vi "linx_analog_okuma_deneme2.vi"() -> ()   [LabVIEW 2017]
uses:
  <vilib>/MakerHub/LINX/Public/Peripherals/Analog/Analog Read 1 Chan.vi
  <vilib>/MakerHub/LINX/Private/Local IO/LinxI2cWrite.vi
  <vilib>/MakerHub/LINX/Public/Utilities/Check Channel.vi
  <vilib>/MakerHub/LINX/Public/Peripherals/Analog/Analog Read N Chans.vi
  <vilib>/MakerHub/LINX/Private/Local IO/LinxAnalogRead.vi
  <vilib>/MakerHub/LINX/Public/Utilities/Open Serial.vi
  <vilib>/MakerHub/LINX/Private/Utilties/Generate Error.vi
  <vilib>/MakerHub/LINX/LMH-LINX.lvlib
panel:
  out "Numeric":dbl
  out "Thermometer":dbl(slide) scale=0.0..100.0
  in  "Serial Port":refnum<visa-resource-name>="N/A"
  in  "stop":bool
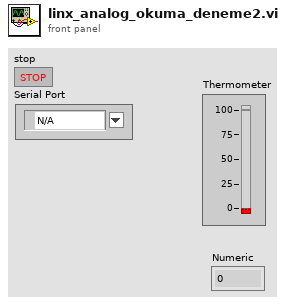
[diagram p1: front panel]
types:
  T1 = typedef "LMH-LINX.lvlib/LINX Ref.ctl" = cluster{"IO":T2, "Interface":T3, "LINX Device Config":T4}
  T2 = typedef "LMH-LINX.lvlib/Platform.ctl" = enum16{"Remote", "Local"}
  T3 = typedef "LMH-LINX.lvlib/Interface.ctl" = enum16{"Serial", "TCP"}
  T4 = typedef "LMH-LINX.lvlib/Device.lvlib/LINX Device Config.ctl" = cluster{"Interface":T3, "COM Port":refnum<visa-resource-name>, "TCP Configuration":T5, "Device Family":u8, "Device ID":u8, "Device Name":string, "TCP Ref":refnum<k5>, "Channels":T6}
  T5 = typedef "LMH-LINX.lvlib/Device.lvlib/TCP Config.ctl" = cluster{"IP Address":string, "Port":u16}
  T6 = typedef "LMH-LINX.lvlib/Channels.ctl" = cluster{"DI":u8[], "DO":u8[], "AI":u8[], "AO":u8[], "PWM":u8[], "QE":u8[], "UART":u8[], "I2C 2":u8[], "SPI":u8[], "CAN":u8[], "Servo":u8[], "AI Ref (V)":dbl, "AI Resolution (Bits)":u8, "AO Ref (V)":dbl, "AO Resolution (Bits)":u8}
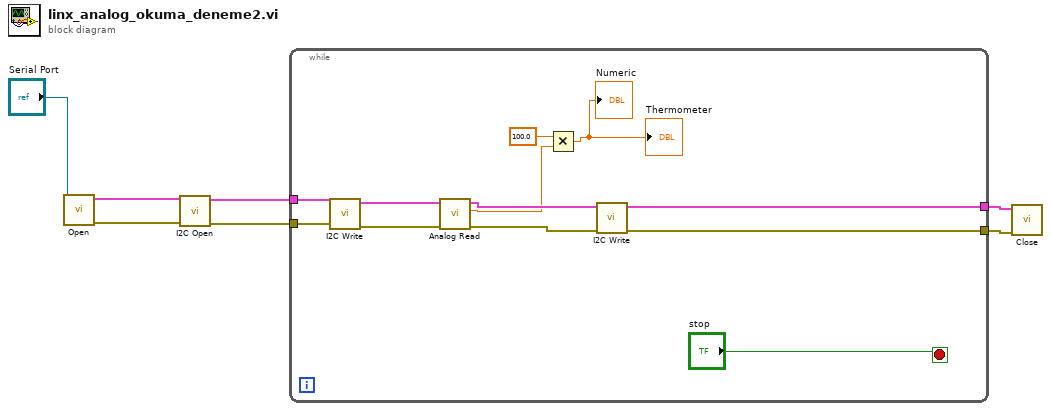
[diagram p0: block diagram]
diagram:
  n1 = call-poly <vilib>:"Open.vi"("Serial Port"="Serial Port") -> ("Error Out"=w5:errorcluster, "LINX Resource"=w6:T1)  [unwired: 8 in, 1 out]
  n2 = call <vilib>:"I2C Open.vi"("Error In"=w5, "LINX Resource"=w6) -> ("Error Out"=w3:errorcluster, "LINX Resource"=w4:T1)  [unwired: 8 in]
  n3 = while {
    tunnel: w4 -> [w17]
    tunnel: w3 -> [w16]
    tunnel: [w15] -> w2
    tunnel: [w14] -> w1
    stop <- "stop" stop-if-true
    n4 = call <vilib>:"I2C Write.vi"("Error In"=w16, "LINX Resource"=w17) -> ("Error Out"=w11:errorcluster, "LINX Resource"=w12:T1)  [unwired: 8 in]
    n5 = call-poly <vilib>:"Analog Read.vi"("Error In"=w11, "LINX Resource"=w12) -> ("Error Out"=w9:errorcluster, "Voltage"=w8:dbl, "LINX Resource"=w10:T1)  [unwired: 6 in, 1 out]
    n6 = Multiply(x=100.0, y=w8) -> (x*y=→"Thermometer" →"Numeric":dbl)
    n7 = call <vilib>:"I2C Write.vi"("Error In"=w9, "LINX Resource"=w10) -> ("Error Out"=w14:errorcluster, "LINX Resource"=w15:T1)  [unwired: 8 in]
  }
  n8 = call <vilib>:"Close.vi"("Error In"=w1, "LINX Resource"=w2) -> ()  [unwired: 9 in, 1 out]
